vi "Get RC Connection Status.vi"(8 "error in (no error)":errorcluster, 11 "Instrument in":refnum<class "Instrument.lvclass">) -> (0 "error out":errorcluster, 2 "RC Connected?":bool, 3 "Instrument out":refnum<class "Instrument.lvclass">)   [LabVIEW 2019, in "Instrument.lvclass"]
uses:
  Instrument.lvclass
  Instrument.lvclass/Instrument.ctl
  RemoteControl/RemoteControl.lvclass/RemoteControl.ctl
  RemoteControl/RemoteControl.lvclass
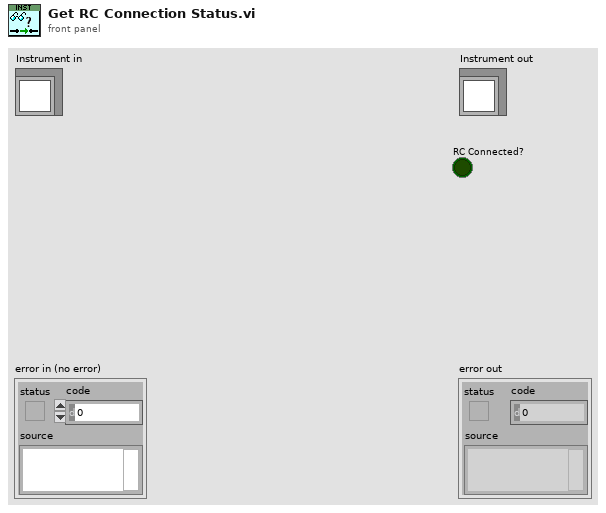
[diagram p1: front panel]
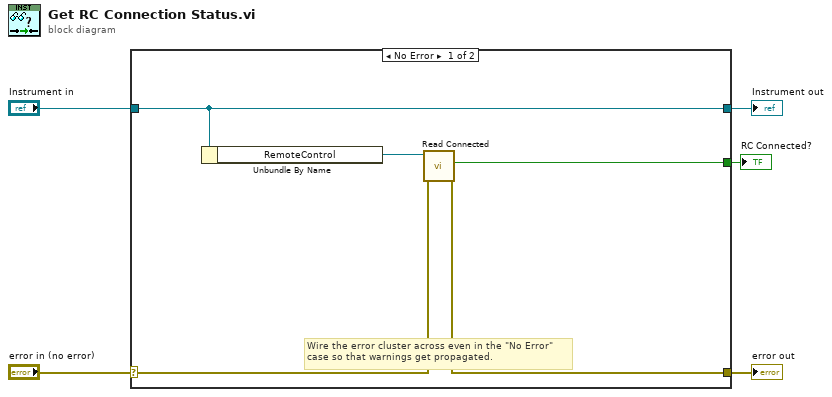
[diagram p0: block diagram]
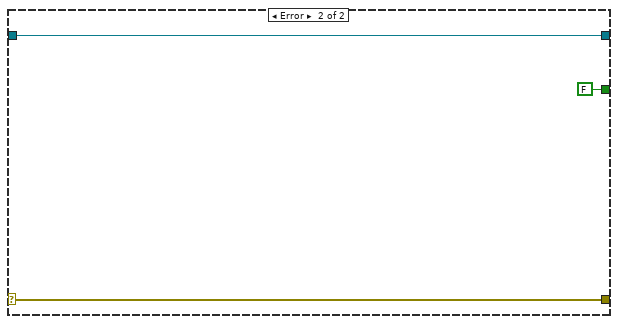
[diagram p2: hidden frame]
diagram:
  n1 = case shown="No Error" "error in (no error)" {
    selector: "error in (no error)" -> [w8 w13]
    tunnel: [w7 w13] -> w4
    tunnel: [w10 w12] -> w2
    tunnel: "Instrument in" -> [w10 w12]
    tunnel: [w6 FALSE ("Connected?")] -> w1
    frame No Error {
      # "Wire the error cluster across even in the \"No Error\"\ncase so that warnings get propagated."
      n2 = Unbundle By Name(w10) -> ("RemoteControl"=w9:refnum<class "RemoteControl.lvclass">)
      n3 = call "Read Connected.vi"("error in (no error)"=w8, "RemoteControl in"=w9) -> ("error out"=w7:errorcluster, "Connected?"=w6:bool)  [unwired: 7 in, 1 out]
    }
    frame Error {
    }
  }
  "error out" <- w4
  "Instrument out" <- w2
  "RC Connected?" <- w1
